vi "SCMP - Write FITS File v2.vi"(1 "FITS Header":T4={"Wavelength (nm)"=530.15, "Exposure (s)"=0.05, "Tuning Delay (ms)"=1000.0, "Beam Type (-1/1)"=1.0, "Tuning Voltages"=[1.111, 2.222, 3.333, 4.444], "Observer"="observer", "Light Shapping Diffuser"=enum."In Beam", "Comment"="", "Data Type"=9, "Mod Cycles"=0, "SCD Calibration Optics"=enum."1 - Polarizer @0, I+Q", "SCD Emission Line Filter"=enum."1-557.6nm", "Cookbook"="", "COMP-S Calibration Wheel"=enum."Dark", "COMP-S Andover Filter Wheel"=enum."530.3nm/HWB 0.34nm (Fe XIV)", "FOV Rotation (deg)"=66.0, "Objective Lens Position (mm)"=0.0, "Occulter size"=0.0, "Time End"=timestamp(3382374145.421875 s since 1904-01-01), "Acc Exposure (s)"=0.0, "Time Stamp Array"=[], "Camera Serial Number"=[], "Camera Temp"=[], "Camera PI (mm)"=[], "Time Start"=timestamp(3382374145.421875 s since 1904-01-01), "Peripherals"={"ILX controler"=FALSE, "Zone temperatures"=FALSE, "Andor"=FALSE, "Andor 2"=FALSE, "PI Stages"=FALSE, "AISAS mechanisms"=FALSE, "AISAS Mech.lvclass"=refnum, "Zone temp ref"=variant, "FWs"=FALSE}, "FITS paths"=[], "Cameras"=enum."Andor", "load preset cbk"=FALSE, "periodic check count"=0} {"Camera PI (mm)" format="%_3g"; "Acc Exposure (s)" format="%^.3g"; "Occulter size" format="%.2f"; "Objective Lens Position (mm)" min=70.0 max=152.0 format="%.2f"; "FOV Rotation (deg)" format="%.1f"; "Data Type" items=["LIVE", "DARK", "FLAT", "CALI", "OBSE", "ABSO", "AURE", "TARG", "OBJE", "HOLE", "OREX", "THRO", "CHIP"]; "Exposure (s)" format="%^.3g"; "Wavelength (nm)" format="%_6g"}, 2 "Andor":T1={"Handle"=0, "Pixel Encoding"="", "AOI Width"=0, "AOI Height"=0, "AOI Stride"=0, "Row Readout Time"=0.0, "Frame Readout Time"=0.0, "Interframe Time"=0.0, "Semaphore"=refnum, "SerialNumber"="", "Camera Model"="", "Controller ID"="", "Firmware Version"="", "Shutter"="Global", "BDiv"=1, "Time at Synch"=timestamp(3029526000.379448 s since 1904-01-01), "Idx"=0, "PreAmp"="", "Binning"=enum."1x1", "PixelReadoutRate"="", "Exposure (s)"=0.05, "Image Bytes"=0, "Image Pixels"=0, "SpuriousNoiseFilter"=FALSE, "Overlap"=FALSE, "CycleMode"=""} {"Exposure (s)" format="%^.3g"; "Time at Synch" format="%<%H:%M:%S>T"; "Interframe Time" format="%#_3g"; "Frame Readout Time" format="%_3g"; "Row Readout Time" format="%_3g"}, 5 "Data":u32[][][](array[numeric]), 11 "error in":errorcluster, 12 "Image #":i32) -> (4 "FITS Path Out":path=path "G:/SCD Data/Level-0/20141030/20141030.160747.FTS", 6 "<ADU>":dbl[](array[numeric]), 15 "error out":errorcluster)   [LabVIEW 2014]
doc: "Use this template to build a VI to use as a subVI."
uses:
  Controls/SCD - FITS Cluster.ctl
  AISAS/Mech/AISAS Mech.lvclass
  AISAS/Controls/Diffuser.ctl
  Controls/SCD - Calibration Optics Filter Wheel.ctl
  Controls/SCD - EDT - Emission Line Filter Wheel.ctl
  Controls/CoMP-S Controls/Polarization Optics Filter Wheel.ctl
  Controls/CoMP-S Controls/Emission Line Filter Wheel.ctl
  AISAS/Controls/focus.ctl
  Controls/peripherals.ctl
  Controls/Cameras select.ctl
  Camera/Andor Neo Info.ctl
  Controls/beaning.ctl
panel:
  out "size(s)":i32
  in  "A":u32[][](array[numeric])
  in  "D":u32[][](array[numeric])
  in  "C":u32[][](array[numeric])
  in  "B":u32[][](array[numeric])
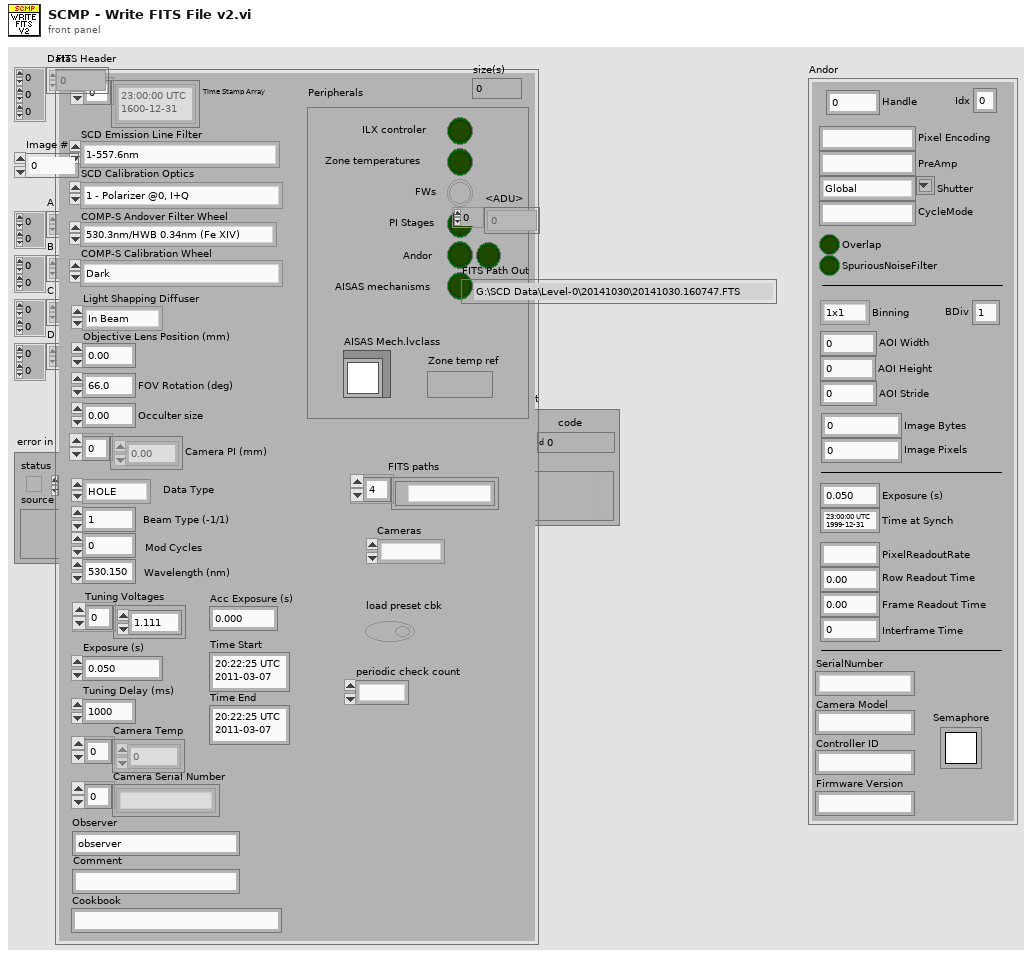
[diagram p1: front panel]
types:
  T1 = typedef "Andor Neo Info.ctl" = cluster{"Handle":i32, "Pixel Encoding":string, "AOI Width":i32, "AOI Height":i32, "AOI Stride":i32, "Row Readout Time":dbl, "Frame Readout Time":dbl, "Interframe Time":dbl, "Semaphore":T2, "SerialNumber":string, "Camera Model":string, "Controller ID":string, "Firmware Version":string, "Shutter":string, "BDiv":u8, "Time at Synch":timestamp, "Idx":i32, "PreAmp":string, "Binning":T3, "PixelReadoutRate":string, "Exposure (s)":dbl, "Image Bytes":i64, "Image Pixels":i64, "SpuriousNoiseFilter":bool, "Overlap":bool, "CycleMode":string}
  T2 = typedef "Semaphore RefNum" = refnum<k1>
  T3 = typedef "beaning.ctl" = enum16{"1x1", "2x2", "3x3", "4x4", "8x8"}
  T4 = typedef "SCD - FITS Cluster.ctl" = cluster{"Wavelength (nm)":dbl, "Exposure (s)":dbl, "Tuning Delay (ms)":dbl, "Beam Type (-1/1)":dbl, "Tuning Voltages":dbl[], "Observer":string, "Light Shapping Diffuser":T5, "Comment":string, "Data Type":u16, "Mod Cycles":u16, "SCD Calibration Optics":T6, "SCD Emission Line Filter":T7, "Cookbook":string, "COMP-S Calibration Wheel":T8, "COMP-S Andover Filter Wheel":T9, "FOV Rotation (deg)":dbl, "Objective Lens Position (mm)":T10, "Occulter size":dbl, "Time End":timestamp, "Acc Exposure (s)":dbl, "Time Stamp Array":timestamp[], "Camera Serial Number":string[], "Camera Temp":dbl[], "Camera PI (mm)":dbl[], "Time Start":timestamp, "Peripherals":T11, "FITS paths":path[], "Cameras":T12, "load preset cbk":bool, "periodic check count":i32}
  T5 = typedef "Diffuser.ctl" = enum16{"Out of Beam", "In Beam"}
  T6 = typedef "SCD - Calibration Optics Filter Wheel.ctl" = enum16{"1 - Polarizer @0, I+Q", "2 - Polarizer @90, I-Q", "3 - Polarizer @45, I+U", "4 - Polarizer @135, I-U", "5 - Polarizer @0, Retarder @45, I+V", "6 - Polarizer @0, Retarder @135, I-V", "7 - Dark", "8 - Clear", "9 - N/A"}
  T7 = typedef "SCD - EDT - Emission Line Filter Wheel.ctl" = enum16{"1-557.6nm", "2-587.6nm", "3-589.6nm", "4-630.2nm", "5-656.4nm", "6-849.8nm", "7-854.2nm", "8-866.2nm", "9-1083.0nm"}
  T8 = typedef "Polarization Optics Filter Wheel.ctl" = enum16{"Dark", "Clear", "Exchange Lens", "Polarizer @0, I+Q", "Polarizer @90, I-Q", "Polarizer @45, I+U", "Polarizer @135, I-U", "Polarizer @0, Retarder @45, I+V", "Polarizer @0, Retarder @135, I-V"}
  T9 = typedef "Emission Line Filter Wheel.ctl" = enum16{"530.3nm/HWB 0.34nm (Fe XIV)", "587.6nm/HBW 0.44nm (He I D3)", "637.5nm/HBW 0.53nm (Fe X)", "656.3nm/HBW 0.57nm (H-Alpha)", "789.2nm/HBW 0.85nm (Fe XI)", "854.2nm/HBW 1.01nm (Ca I)", "1074.7nm/HBW 2.34nm (Fe XIII)", "1079.8nm/HBW 1.64nm (Fe XIII)", "1083.0nm/HBW 1.66nm (He I)"}
  T10 = typedef "focus.ctl" = dbl
  T11 = typedef "peripherals.ctl" = cluster{"ILX controler":bool, "Zone temperatures":bool, "Andor":bool, "Andor 2":bool, "PI Stages":bool, "AISAS mechanisms":bool, "AISAS Mech.lvclass":refnum<class "AISAS Mech.lvclass">, "Zone temp ref":variant, "FWs":bool}
  T12 = typedef "Cameras select.ctl" = enum16{"Andor", "GDR"}
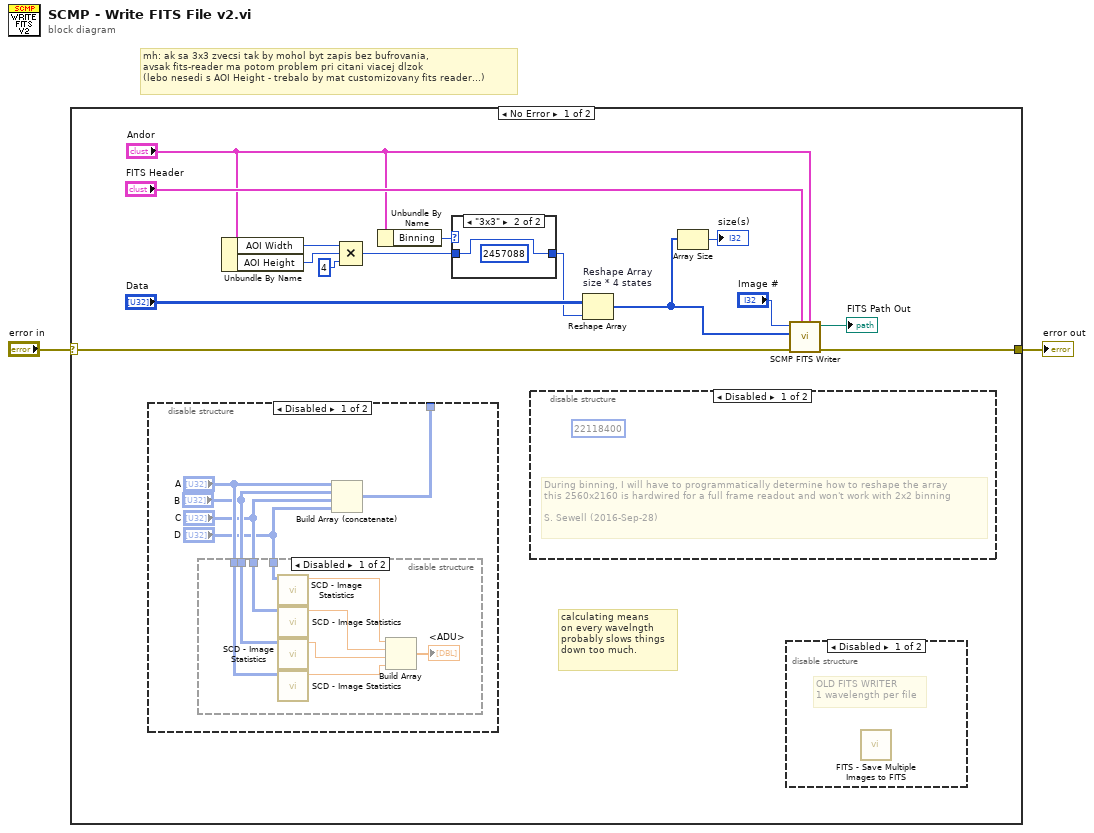
[diagram p0: block diagram]
diagram:
  # "mh: ak sa 3x3 zvecsi tak by mohol byt zapis bez bufrovania, \navsak fits-reader ma potom problem pri citani viacej dlzok\n(lebo nesedi s AOI Height - trebalo by mat customizovany fits reader...)"
  n1 = case shown="No Error" "error in" {
    selector: "error in" -> [w16 w34]
    tunnel: [w17 w34] -> w1
    frame No Error {
      # "calculating means\non every wavelngth\nprobably slows things\ndown too much."
      n2 = disable-structure shown="Disabled" {
        disable-tunnel: [w24 _] -> _
        frame Disabled {
          n3 = disable-structure shown="Disabled" {
            disable-tunnel: "A" -> [w33 _]
            disable-tunnel: "B" -> [w32 _]
            disable-tunnel: "C" -> [w31 _]
            disable-tunnel: "D" -> [w30 _]
            frame Disabled {
              n4 = call "SCD - Image Statistics.vi"("I32 Image"=w30) -> ("mean"=w29:dbl)  [unwired: 9 in, 1 out]
              n5 = call "SCD - Image Statistics.vi"("I32 Image"=w31) -> ("mean"=w28:dbl)  [unwired: 9 in, 1 out]
              n6 = call "SCD - Image Statistics.vi"("I32 Image"=w32) -> ("mean"=w27:dbl)  [unwired: 9 in, 1 out]
              n7 = call "SCD - Image Statistics.vi"("I32 Image"=w33) -> ("mean"=w26:dbl)  [unwired: 9 in, 1 out]
              n8 = Build Array(w29, w28, w27, w26) -> (→"<ADU>":dbl[])
            }
            frame Enabled {
            }
          }
          n9 = Build Array (concatenate)("A", "B", "C", "D") -> (w24:u32[][])
        }
        frame Enabled {
        }
      }
      n10 = Unbundle By Name("Andor") -> ("AOI Width"=w12:i32, "AOI Height"=w11:i32)
      n11 = Compound Arithmetic op=MULTIPLY(w12, w11, i64 4 ("value")) -> (w7:i64)
      n12 = Unbundle By Name("Andor") -> ("Binning"=w8:T3)
      n13 = case shown="\"3x3\"" w8 {
        tunnel: w7 -> [w18 w19]
        tunnel: [w18 w19] -> w5
        frame "1x1", Default {
        }
        frame "3x3" {
          (unwired) 2457088 ("dimension size")
        }
      }
      n14 = disable-structure shown="Disabled" {
        frame Disabled {
          (unwired) 22118400 ("dimension size")
          # "During binning, I will have to programmatically determine how to reshape the array\nthis 2560x2160 is hardwired for a full frame readout and won't work with 2x2 binning\n\nS. Sewell (2016-Sep-28)"
        }
        frame Enabled {
        }
      }
      n15 = Reshape Array "Reshape Array\nsize * 4 states"("Data", w5) -> (w4:u32[])
      n16 = Array Size(array=w4) -> (size(s)=→"size(s)":i32)
      n17 = disable-structure shown="Disabled" {
        frame Disabled {
          # "OLD FITS WRITER\n1 wavelength per file"
          n18 = call "FITS - Save Multiple Images to FITS.vi"() -> ()  [unwired: 9 in, 3 out]
        }
        frame Enabled {
        }
      }
      n19 = call "SCMP FITS Writer.vi"("Andor"="Andor", "FITS Cluster"="FITS Header", "error in"=w16, "Image Vector"=w4, "Wavelength (0..n)"="Image #") -> ("error out"=w17:errorcluster, "Current FITS Path"=→"FITS Path Out":path)  [unwired: 5 in]
    }
    frame Error {
    }
  }
  "error out" <- w1
